vi "value to ring (SequenceNumberInit).vi"(11 "value":string) -> (3 "SequenceNumberInit":T1=65535 items=["FDX_TX_FRAME_SEQ_INIT_AUTO"=65535, "FDX_TX_FRAME_SEQ_OFF"=65533])   [LabVIEW 2020, in "AIM ARINC 664 Import.lvlib"]
uses:
  AIM ARINC 664 Import.lvlib
  _typedefs/frame_tx_generic_seqNumberInit.ctl
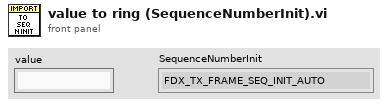
[diagram p1: front panel]
types:
  T1 = typedef "AIM ARINC 664 Import.lvlib/frame_tx_generic_seqNumberInit.ctl" = i32
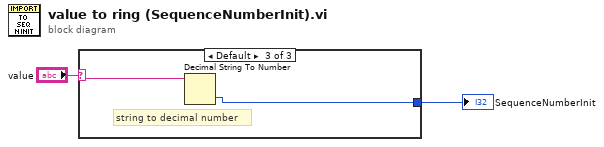
[diagram p0: block diagram]
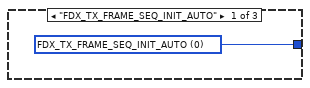
[diagram p2: hidden frame]
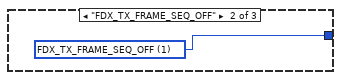
[diagram p3: hidden frame]
diagram:
  n1 = case shown="Default" "value" {
    selector: "value" -> [_ _ w6]
    tunnel: [w3 w4 w5] -> w1
    frame "FDX_TX_FRAME_SEQ_INIT_AUTO" {
      w3 = T1 0 items=["FDX_TX_FRAME_SEQ_INIT_AUTO", "FDX_TX_FRAME_SEQ_OFF", "Item0255"] ("SequenceNumberInit")
    }
    frame "FDX_TX_FRAME_SEQ_OFF" {
      w4 = T1 1 items=["FDX_TX_FRAME_SEQ_INIT_AUTO", "FDX_TX_FRAME_SEQ_OFF", "Item0255"] ("SequenceNumberInit")
    }
    frame Default {
      # "string to decimal number"
      n2 = Decimal String To Number(string=w6) -> (number=w5:i32)  [unwired: 2 in, 1 out]
    }
  }
  "SequenceNumberInit" <- w1
